vi "_save_csv_HAPS_MCU_PhaseCali.vi"(7 "NoteName":string="SingleCh_", 11 "array in":string[][](array[string])) -> (3 "FileName":string)   [LabVIEW 2023, in "HAPS.lvlib"]
uses:
  HAPS.lvlib
  <vilib>/Utility/file.llb/Write Delimited Spreadsheet (string).vi
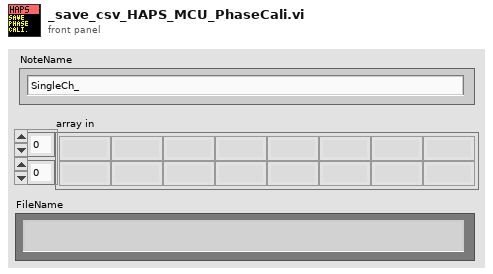
[diagram p1: front panel]
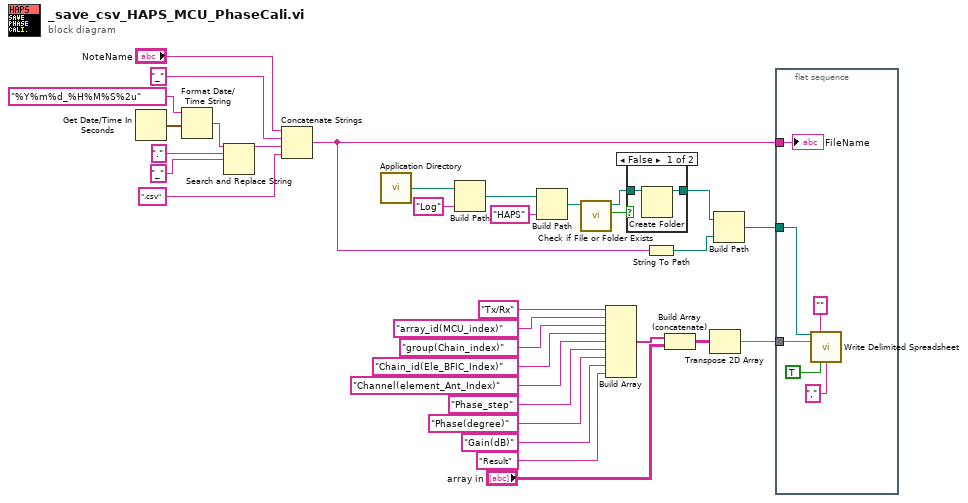
[diagram p0: block diagram]
diagram:
  n1 = Get Date/Time In Seconds() -> (seconds since 1Jan1904=w13:timestamp)
  n2 = Format Date/Time String(time format string (%c)="%Y%m%d_%H%M%S%2u", seconds (now)=w13) -> (date/time string=w11:string)  [unwired: 1 in]
  n3 = Search and Replace String(input string=w11, search string=".", replace string="_") -> (result string=w8:string)  [unwired: 5 in, 3 out]
  n4 = Concatenate Strings("NoteName", "_", w8, ".csv" ("delimiter (\\t)")) -> (w30:string)
  n5 = call <vilib>:"Application Directory.vi"() -> ("Application Directory"=w5:path)
  n6 = Build Path(base path=w5, name or relative path="Log") -> (appended path=w3:path)
  n7 = Build Path(base path=w3, name or relative path="HAPS") -> (appended path=w2:path)
  n8 = call <vilib>:"Check if File or Folder Exists.vi"("path"=w2) -> ("file or folder exists?"=w29:bool, "dup path"=w28:path)  [unwired: 8 in, 1 out]
  n9 = Build Array("Tx/Rx", "array_id(MCU_index)", "group(Chain_index)", "Chain_id(Ele_BFIC_Index)", "Channel(element_Ant_Index)", "Phase_step", "Phase(degree)", "Gain(dB)", "Result") -> (w18:string[])
  n10 = case shown="False" w29 {
    tunnel: w28 -> [w35 w36]
    tunnel: [w34 w36] -> w27
    frame False {
      n11 = Create Folder(path (use dialog)=w35) -> (created path=w34:path)  [unwired: 2 in, 2 out]
    }
    frame True {
    }
  }
  n12 = String To Path(string=w30) -> (path=w32:path)
  n13 = Build Array (concatenate)(w18, "array in") -> (w24:string[][])
  n14 = Transpose 2D Array(2D array=w24) -> (transposed array=w26:string[][])
  n15 = Build Path(base path=w27, name or relative path=w32) -> (appended path=w31:path)
  n16 = flat-sequence {
    tunnel: w31 -> [w41]
    tunnel: w30 -> [w39]
    tunnel: w26 -> [w37]
    frame #0 {
      n17 = call-poly <vilib>:"Write Delimited Spreadsheet.vi"("file path (dialog if empty)"=w41, "format (%s)"="" ("format (%.3f)"), "2D data"=w37, "transpose? (no:F)"=TRUE, "delimiter (\\t)"="," ("delimiter (\\t)")) -> ()  [unwired: 9 in, 2 out]
      "FileName" <- w39
    }
  }
